vi "Pure Pursuit Velocity FF.vi"(5 "kffa":dbl, 7 "kffv":dbl, 8 "dt":dbl format="%0.2f", 9 "Velocity":T1, 10 "Right Desired Velocity":dbl, 11 "Left Desired Velocity":dbl) -> (2 "Right Velocity":dbl, 3 "Left Velocity":dbl)   [LabVIEW 2018, in "Pure Pursuit.lvlib"]
uses:
  Pure Pursuit.lvlib
  Odometry/Typedef/Velocity Data.ctl
  <vilib>/ptbypt/NI_PtbyPt.lvlib
panel:
  in  "reinitialize?":bool
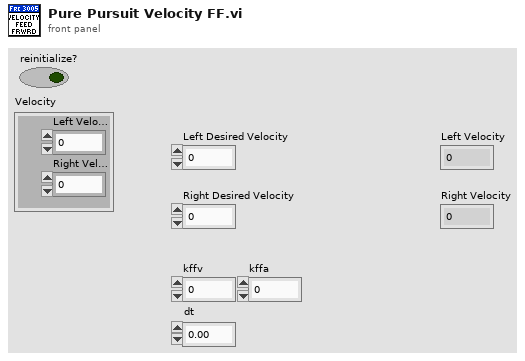
[diagram p1: front panel]
types:
  T1 = typedef "Velocity Data.ctl" = cluster{"Right Velocity Raw":sgl, "Left Velocity Raw":sgl}
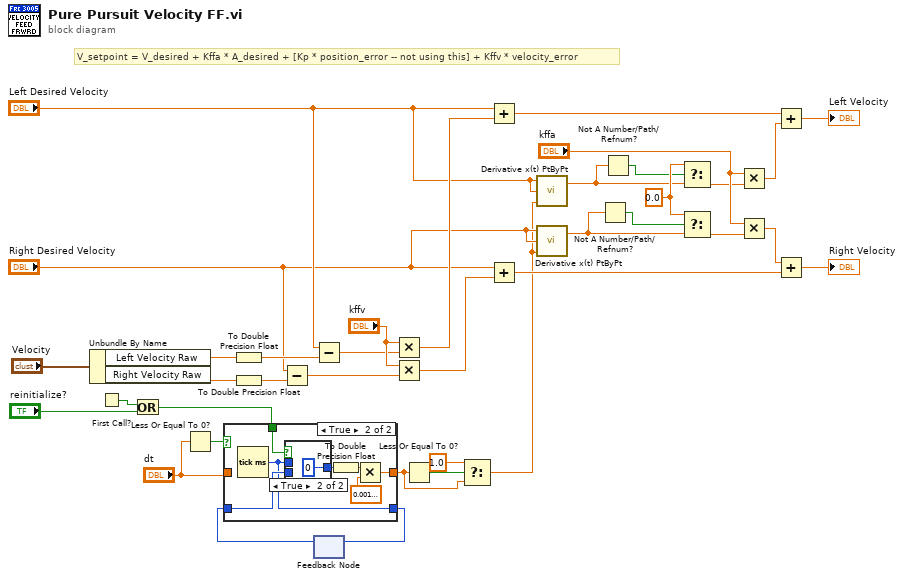
[diagram p0: block diagram]
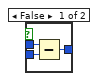
[diagram p3: hidden frame]
diagram:
  w10 = 0.0 ("t")
  # "V_setpoint = V_desired + Kffa * A_desired + [Kp * position_error -- not using this] + Kffv * velocity_error"
  n1 = Unbundle By Name("Velocity") -> ("Left Velocity Raw"=w37:sgl, "Right Velocity Raw"=w35:sgl)
  n2 = First Call?() -> (First Call?: T/F=w17:bool)
  n3 = Or(x=w17, y="reinitialize?") -> (x .or. y?=w18:bool)
  n4 = Less Or Equal To 0?(x="dt") -> (x <= 0?=w15:bool)
  n5 = To Double Precision Float(number=w37) -> (double precision float=w36:dbl)
  n6 = To Double Precision Float(number=w35) -> (double precision float=w34:dbl)
  n7 = Subtract(x="Right Desired Velocity", y=w34) -> (x-y=w22:dbl)
  n8 = Subtract(x="Left Desired Velocity", y=w36) -> (x-y=w23:dbl)
  n9 = feedback #1() -> (w20:u32)  [unwired: 1 in]
  n10 = case shown="True" w15 {
    tunnel: [w39 w43] -> w2
    tunnel: w20 -> [w38 w42]
    tunnel: [w38 w41] -> w21
    tunnel: "dt" -> [w39 _]
    tunnel: w18 -> [_ w40]
    frame False {
    }
    frame True {
      n11 = Tick Count (ms)() -> (millisecond timer value=w41:u32)
      n12 = case shown="True" w40 {
        tunnel: [w49 u32 0] -> w45
        tunnel: w42 -> [w48 _]
        tunnel: w41 -> [w47 _]
        frame False {
          n13 = Subtract(x=w47, y=w48) -> (x-y=w49:u32)
        }
        frame True {
        }
      }
      n14 = To Double Precision Float(number=w45) -> (double precision float=w44:dbl)
      n15 = Multiply(x=w44, y=0.0010000000474974513) -> (x*y=w43:dbl)
    }
  }
  n16 = feedback-in #1(w21) -> ()
  n17 = Multiply(x="kffv", y=w23) -> (x*y=w30:dbl)
  n18 = Multiply(x="kffv", y=w22) -> (x*y=w29:dbl)
  n19 = Less Or Equal To 0?(x=w2) -> (x <= 0?=w4:bool)
  n20 = Select(t=1.0, s=w4, f=w2) -> (s? t:f=w5:dbl)
  n21 = Add(x="Left Desired Velocity", y=w30) -> (x+y=w33:dbl)
  n22 = Add(x="Right Desired Velocity", y=w29) -> (x+y=w31:dbl)
  n23 = call <vilib>:"Derivative x(t) PtByPt.vi"("dt"=w5, "initial condition"="Left Desired Velocity", "x"="Left Desired Velocity") -> ("dx/dt"=w9:dbl)  [unwired: 1 in, 1 out]
  n24 = call <vilib>:"Derivative x(t) PtByPt.vi"("dt"=w5, "initial condition"="Right Desired Velocity", "x"="Right Desired Velocity") -> ("dx/dt"=w12:dbl)  [unwired: 1 in, 1 out]
  n25 = Not A Number/Path/Refnum?(number/path/refnum=w12) -> (NaN/Path/Refnum?=w11:bool)
  n26 = Not A Number/Path/Refnum?(number/path/refnum=w9) -> (NaN/Path/Refnum?=w8:bool)
  n27 = Select(t=w10, s=w8, f=w9) -> (s? t:f=w14:dbl)
  n28 = Select(t=w10, s=w11, f=w12) -> (s? t:f=w13:dbl)
  n29 = Multiply(x="kffa", y=w14) -> (x*y=w26:dbl)
  n30 = Multiply(x="kffa", y=w13) -> (x*y=w24:dbl)
  n31 = Add(x=w33, y=w26) -> (x+y=→"Left Velocity":dbl)
  n32 = Add(x=w24, y=w31) -> (x+y=→"Right Velocity":dbl)
